vi "TTA_Instrument_Cluster.vi"() -> ()   [LabVIEW 2016]
panel:
  in  "Instrument Cluster":T1
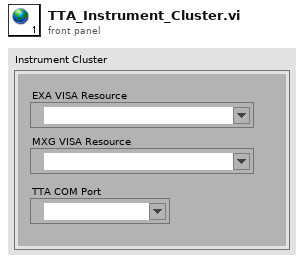
[diagram p1: front panel]
types:
  T1 = cluster{"EXA VISA Resource":refnum<visa-resource-name>, "MXG VISA Resource":refnum<visa-resource-name>, "TTA COM Port":refnum<visa-resource-name>}
diagram:
